vi "U16 to U8.vi"(8 "error in (no error)":errorcluster, 9 "Image 16 in":T1, 10 "Image 8 in":T1, 11 "Cascade in":refnum<class "Cascade.lvclass">) -> (0 "error out":errorcluster, 2 "Image 8 out":T1, 3 "Cascade out":refnum<class "Cascade.lvclass">)   [LabVIEW 2012, in "Cascade.lvclass"]
uses:
  Cascade.lvclass
  <vilib>/vision/Image Controls.llb/IMAQ Image.ctl
  Cascade.lvclass/Cascade.ctl
  <vilib>/vision/NI_Vision_Development_Module.lvlib
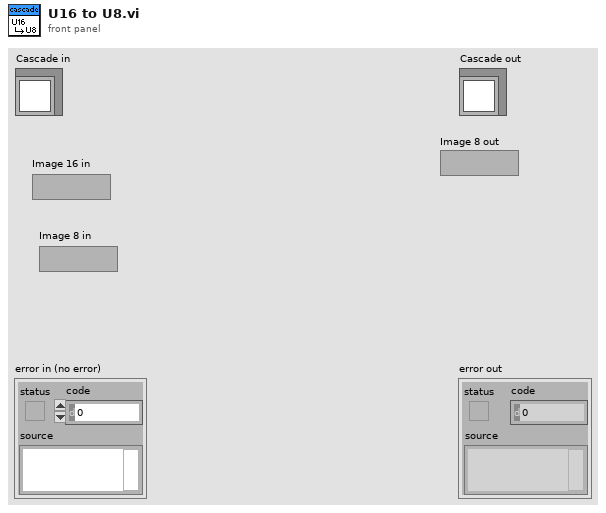
[diagram p1: front panel]
types:
  T1 = typedef "IMAQ Image.ctl" = refnum<image>
  T2 = typedef "Image Type" = u32
  T3 = cluster{"Mean Value":sgl, "Standard Variation":sgl, "Minimal Value":sgl, "Maximal Value":sgl, "Area (calibrated)":sgl, "Area (pixels)":u32, "%":sgl, "Calibration Valid":bool}
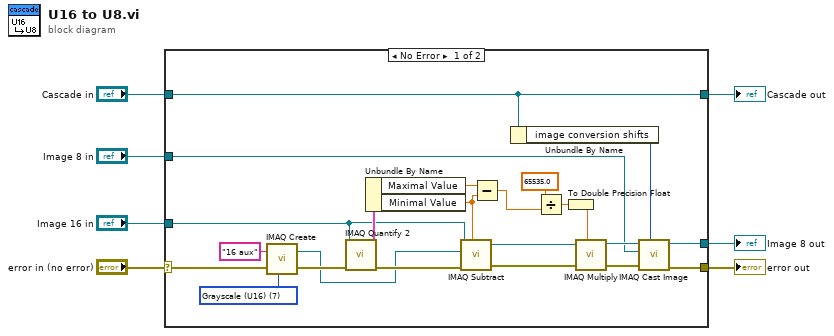
[diagram p0: block diagram]
diagram:
  n1 = case shown="No Error" "error in (no error)" {
    selector: "error in (no error)" -> [w13 w33]
    tunnel: [w12 w33] -> w6
    tunnel: [w30 w32] -> w4
    tunnel: "Cascade in" -> [w30 w32]
    tunnel: "Image 16 in" -> [w20 _]
    tunnel: "Image 8 in" -> [w10 w31]
    tunnel: [w8 w31] -> w1
    frame No Error {
      w18 = T2 7 items=["Grayscale (U8)", "Grayscale (I16)", "Grayscale (SGL)", "Complex (CSG)", "RGB (U32)", "HSL (U32)", "RGB (U64)", "Grayscale (U16)"] ("Image Type")
      n2 = call "IMAQ Create"("Image Name"="16 aux", "Image Type"=w18, "error in (no error)"=w13) -> ("New Image"=w11:T1, "error out"=w17:errorcluster)  [unwired: 2 in]
      n3 = call "IMAQ Quantify 2"("error in (no error)"=w17, "Image"=w20) -> ("error out"=w16:errorcluster, "Global Report"=w29:T3)  [unwired: 7 in, 1 out]
      n4 = Unbundle By Name(w29) -> ("Maximal Value"=w24:sgl, "Minimal Value"=w23:sgl)
      n5 = call "IMAQ Subtract"("Image Src A"=w20, "Constant"=w23, "Image Dst"=w11, "error in (no error)"=w16) -> ("Image Dst Out"=w25:T1, "error out"=w15:errorcluster)  [unwired: 3 in]
      n6 = Subtract(x=w24, y=w23) -> (x-y=w22:sgl)
      n7 = Unbundle By Name(w30) -> ("image conversion shifts"=w9:i32)
      n8 = Divide(x=sgl 65535.0, y=w22) -> (x/y=w27:sgl)
      n9 = To Double Precision Float(number=w27) -> (double precision float=w26:dbl)
      n10 = call "IMAQ Multiply"("Image Src A"=w25, "Constant"=w26, "error in (no error)"=w15) -> ("Image Dst Out"=w21:T1, "error out"=w14:errorcluster)  [unwired: 4 in]
      n11 = call "IMAQ Cast Image"("# Shifts"=w9, "error in (no error)"=w14, "Image Dst"=w10, "Image Src"=w21) -> ("error out"=w12:errorcluster, "Image Dst Out"=w8:T1)  [unwired: 6 in]
    }
    frame Error {
    }
  }
  "error out" <- w6
  "Cascade out" <- w4
  "Image 8 out" <- w1
